vi "getTimeXml.vi"(8 "error in (no error)":errorcluster, 11 "ScriptEvent in":refnum<class "ScriptEvent.lvclass">) -> (0 "error out":errorcluster, 2 "timeXML":refnum<class "xmlNode.lvclass">, 3 "ScriptEvent out":refnum<class "ScriptEvent.lvclass">)   [LabVIEW 2011, in "Tools.lvlib" / "Scripting.lvlib" / "ScriptEvent.lvclass"]
uses:
  ScriptEvent.lvclass
  xmlNode/xmlNode.lvclass
  ScriptEvent.lvclass/ScriptEvent.ctl
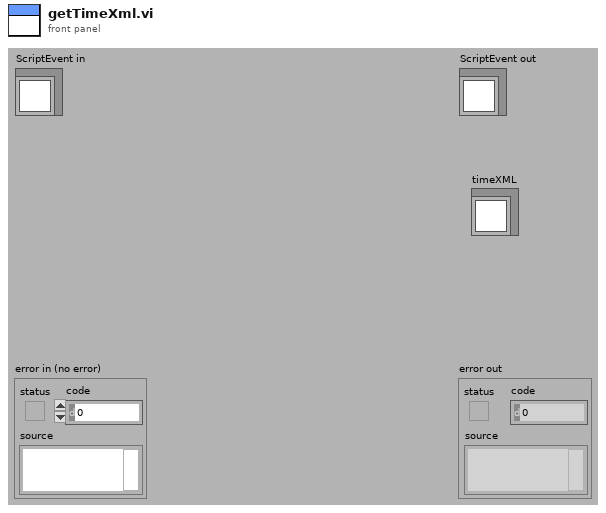
[diagram p1: front panel]
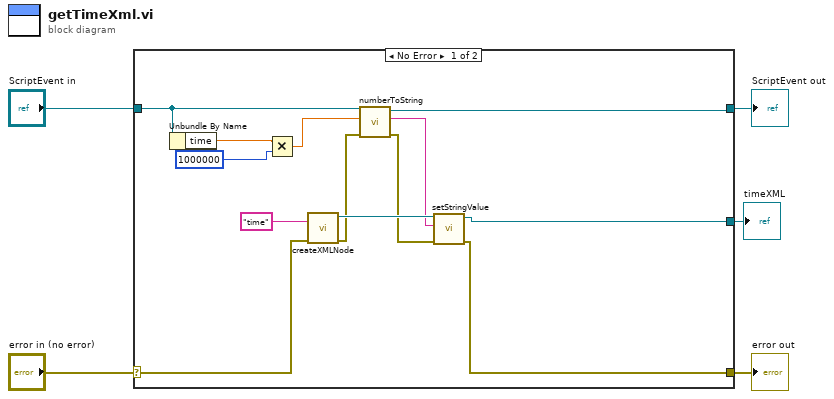
[diagram p0: block diagram]
diagram:
  n1 = case shown="No Error" "error in (no error)" {
    selector: "error in (no error)" -> [w16 w20]
    tunnel: [w15 w20] -> w4
    tunnel: [w7 w19] -> w2
    tunnel: "ScriptEvent in" -> [w8 w19]
    tunnel: [w14 _] -> w1
    frame No Error {
      n2 = Unbundle By Name(w8) -> ("time"=w13:dbl)
      n3 = Multiply(x=w13, y=1000000) -> (x*y=w11:dbl)
      n4 = call "createXMLNode.vi"("error in (no error)"=w16, "name"="time") -> ("error out"=w9:errorcluster, "xmlNode out"=w17:refnum<class "xmlNode.lvclass">)  [unwired: 8 in]
      n5 = call "numberToString.vi"("error in (no error)"=w9, "Numeric"=w11, "ScriptEvent in"=w8) -> ("error out"=w6:errorcluster, "String"=w10:string, "ScriptEvent out"=w7:refnum<class "ScriptEvent.lvclass">)  [unwired: 6 in]
      n6 = call-dynamic "setStringValue.vi"("error in (no error)"=w6, "stringValue"=w10, "xmlNode.lvclass in"=w17) -> ("error out"=w15:errorcluster, "xmlNode.lvclass out"=w14:refnum<class "xmlNode.lvclass">)  [unwired: 7 in]
    }
    frame Error {
    }
  }
  "error out" <- w4
  "ScriptEvent out" <- w2
  "timeXML" <- w1
